vi "yokogawa file save to file_test.vi"() -> ()   [LabVIEW 2011]
panel:
  in  "Error In":errorcluster
  in  "Trace (0:A)":enum16{"A", "B", "C"}(ring)
  in  "VISA session":refnum<visa-resource-name>="GPIB0::1::INSTR"
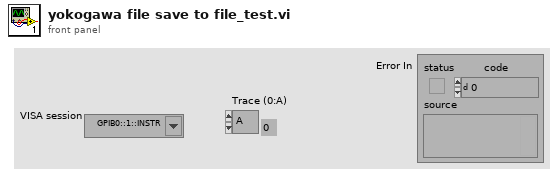
[diagram p1: front panel]
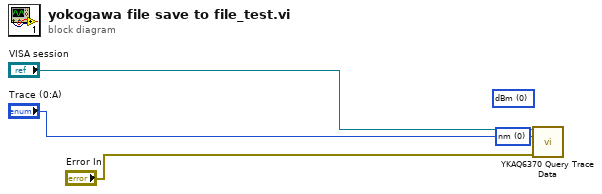
[diagram p0: block diagram]
diagram:
  (unwired) u16 0 items=["nm", "THz", "cm-1"] ("Unit X")
  (unwired) u16 0 items=["dBm", "W", "dBm/nm", "W/nm", "W", "dBm/nm", "W/nm"] ("Unit Y")
  n1 = call <instrlib>:"YKAQ6370 Query Trace Data.vi"("VISA resource name"="VISA session", "Select Trace  (0: Trace A)"="Trace (0:A)", "error in (no error)"="Error In") -> ()  [unwired: 7 in, 6 out]
